vi "Get Plugin Parameter.vi"(7 "Plugin":string, 8 "error in (no error)":errorcluster, 9 "Default Value":string, 10 "Name":string, 11 "Configuration Manager in":refnum<class "Configuration Manager.lvclass">) -> (0 "error out":errorcluster, 2 "Value":string, 3 "Configuration Manager out":refnum<class "Configuration Manager.lvclass">)   [LabVIEW 2020, in "Configuration Manager.lvclass"]
uses:
  Configuration Manager.lvclass
  Configuration Manager.lvclass/Configuration Manager.ctl
  <vilib>/Utility/config.llb/Read Key (String).vi
  <vilib>/Utility/config.llb/Write Key (String).vi
  <vilib>/Utility/config.llb/NI_LVConfig.lvlib
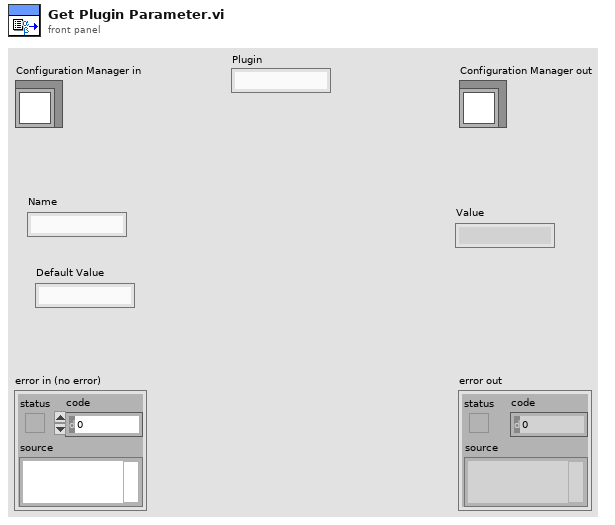
[diagram p1: front panel]
types:
  T1 = typedef "NI_LVConfig.lvlib/Config Data RefNum.ctl" = refnum<k1>
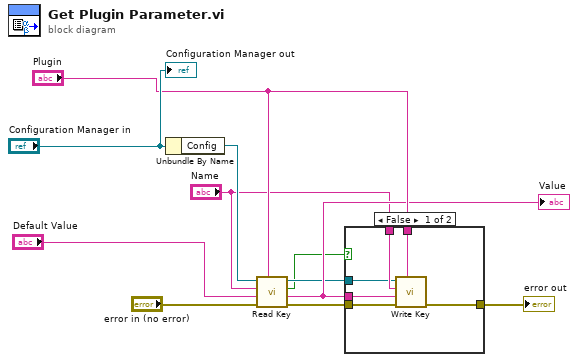
[diagram p0: block diagram]
diagram:
  n1 = Unbundle By Name("Configuration Manager in") -> ("Config"=w10:T1)
  n2 = call-poly <vilib>:"Read Key.vi"("section"="Plugin", "error in (no error)"="error in (no error)", "default value"="Default Value", "key"="Name", "refnum"=w10) -> ("error out"=w8:errorcluster, "value"=w4:string, "found?"=w1:bool, "refnum out"=w2:T1)  [unwired: 3 in]
  "Value" <- w4
  n3 = case shown="False" w1 {
    tunnel: w8 -> [w17 w18]
    tunnel: [w16 w18] -> w5
    tunnel: w4 -> [w15 _]
    tunnel: "Name" -> [w14 _]
    tunnel: "Plugin" -> [w13 _]
    tunnel: w2 -> [w12 _]
    frame False {
      n4 = call-poly <vilib>:"Write Key.vi"("section"=w13, "error in (no error)"=w17, "value"=w15, "key"=w14, "refnum"=w12) -> ("error out"=w16:errorcluster)  [unwired: 4 in, 2 out]
    }
    frame True {
    }
  }
  "error out" <- w5
  "Configuration Manager out" <- "Configuration Manager in"
